vi "SMU Measurement.vi"() -> ()   [LabVIEW 2021]
doc: "Demonstrates how to use the DC Voltage Output Function to force an output voltage. This example initializes a session, configures the Output Function, Sense, Autorange, Voltage Level and Current Limit, initiates generation, waits for a specified delay, and measures the voltage and current output. This example uses Single Point source mode."
uses:
  <instrlib>/niDMM/nidmm.llb/niDMM Resolution in Digits.ctl
  <instrlib>/niDMM/nidmm.llb/niDMM Function.ctl
  <instrlib>/niDCPower/nidcpower.llb/niDCPower Output Function.ctl
  <instrlib>/niDCPower/nidcpower.llb/niDCPower Source Mode.ctl
  <instrlib>/niDMM/nidmm.llb/niDMM Configure Measurement Digits.vi
panel:
  out "SMU Measurement":dbl format="%.6p"
  in  "SMU DMM":refnum<k15>="Dev1"
  in  "SMU DMM Measurement":T1
  out "SMU DMM Resolution":dbl caption="SMU Absolute Resolution" format="%#_3p"
  in  "SMU Resolution in Digits":T2=5.5 items=["3 1/2"=3.5, "4 1/2"=4.5, "5 1/2"=5.5, "6 1/2"=6.5, "7 1/2"=7.5]
  in  "Load SMU":refnum<k15>="Dev1"
  in  "Load SMU Channel":string="0"
  out "Load SMU Current":dbl
  out "Load SMU Voltage":dbl
  in  "error in":errorcluster
  out "error out":errorcluster
  out "Voltage Measurement":dbl caption="Vin SMU Voltage"
  out "Current Measurement":dbl caption="Vin SMU Current"
  in  "Current Limit":dbl=0.01 format="%.3p"
  in  "Voltage Level":dbl=2.0 format="%.5p"
  in  "Vin SMU Channel":string="0"
  in  "Vin SMU":refnum<k15>="Dev1"
  # "Overview: Demonstrates how to use the DC Voltage Output Function to force an output voltage.  \nThis example initializes a session; configures the Output Function, Voltage Level and Current Limit; \ninitiates generation; waits for a specified delay; and measures the voltage and current output. \nRequirements: NI-DCPower\nInstructions:\n1. Select the appropriate device in the Resource Name control.\n2. Configure the parameters of the DC Voltage signal you'd like to output.\n3. Run the VI."
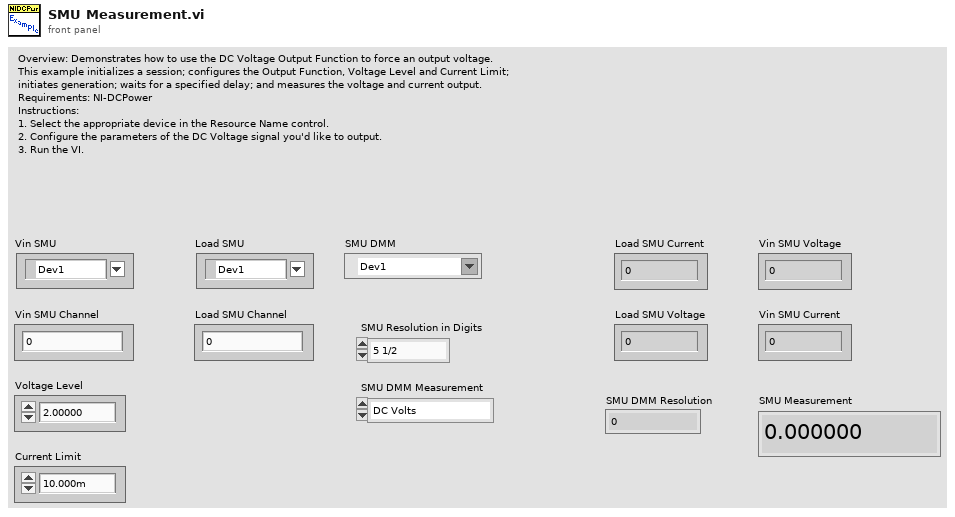
[diagram p1: front panel]
types:
  T1 = typedef "niDMM Function.ctl" = enum16{"DC Volts", "AC Volts", "DC Current", "AC Current", "2-wire Resistance", "4-wire Resistance", "Diode", "Frequency", "Period", "AC Volts DC Coupled", "Capacitance", "Inductance", "Temperature"}
  T2 = typedef "niDMM Resolution in Digits.ctl" = dbl
  T3 = typedef "niDCPower Output Function.ctl" = i32
  T4 = typedef "niDCPower Source Mode.ctl" = i32
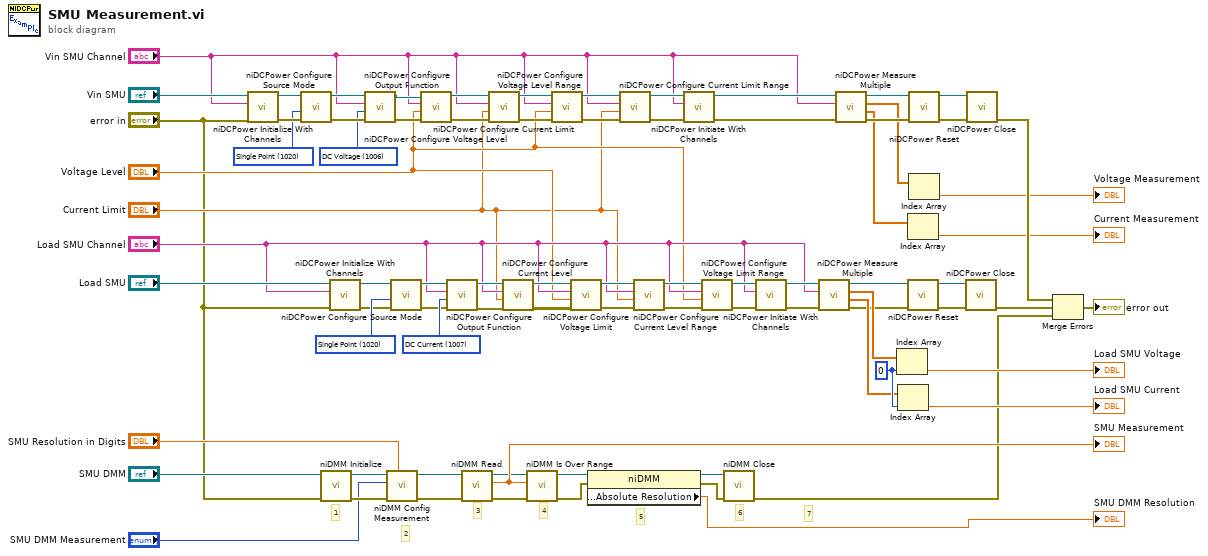
[diagram p0: block diagram]
diagram:
  w51 = T3 1007 items=["DC Voltage"=1006, "DC Current"=1007, "Pulse Voltage"=1049, "Pulse Current"=1050] ("output function")
  w42 = 0 ("index")
  w33 = T4 1020 items=["Single Point"=1020, "Sequence"=1021] ("source mode")
  w57 = T3 1006 items=["DC Voltage"=1006, "DC Current"=1007, "Pulse Voltage"=1049, "Pulse Current"=1050] ("output function")
  w70 = T4 1020 items=["Single Point"=1020, "Sequence"=1021] ("source mode")
  # "2"
  # "1"
  # "7"
  # "6"
  # "5"
  # "4"
  # "3"
  n1 = call <instrlib>:"niDCPower Initialize With Channels.vi"("error in (no error)"="error in", "channels"="Vin SMU Channel", "resource name"="Vin SMU") -> ("error out"=w74:errorcluster, "instrument handle out"=w73:refnum<k15>)  [unwired: 2 in, 5 out]
  n2 = call <instrlib>:"niDCPower Configure Source Mode.vi"("error in (no error)"=w74, "source mode"=w70, "instrument handle"=w73) -> ("error out"=w72:errorcluster, "instrument handle out"=w71:refnum<k15>)  [unwired: 7 out]
  n3 = call <instrlib>:"niDMM Initialize.vi"("error in (no error)"="error in", "Instrument Descriptor"="SMU DMM") -> ("error out"=w10:errorcluster, "instrument handle out"=w11:refnum<k15>)  [unwired: 8 in]
  n4 = call <instrlib>:"niDCPower Initialize With Channels.vi"("error in (no error)"="error in", "channels"="Load SMU Channel", "resource name"="Load SMU") -> ("error out"=w29:errorcluster, "instrument handle out"=w30:refnum<k15>)  [unwired: 2 in, 5 out]
  n5 = call <instrlib>:"niDCPower Configure Output Function.vi"("error in (no error)"=w72, "output function"=w57, "channel name"="Vin SMU Channel", "instrument handle"=w71) -> ("error out"=w58:errorcluster, "instrument handle out"=w59:refnum<k15>)  [unwired: 6 out]
  n6 = call-poly <instrlib>:"niDMM Config Measurement.vi"("Resolution in Digits"="SMU Resolution in Digits", "error in (no error)"=w10, "Function"="SMU DMM Measurement", "instrument handle"=w11) -> ("error out"=w4:errorcluster, "instrument handle out"=w5:refnum<k15>)  [unwired: 6 in]
  n7 = call <instrlib>:"niDCPower Configure Source Mode.vi"("error in (no error)"=w29, "source mode"=w33, "instrument handle"=w30) -> ("error out"=w31:errorcluster, "instrument handle out"=w32:refnum<k15>)  [unwired: 7 out]
  n8 = call <instrlib>:"niDCPower Configure Voltage Level.vi"("error in (no error)"=w58, "voltage level"="Voltage Level", "channel name"="Vin SMU Channel", "instrument handle"=w59) -> ("error out"=w77:errorcluster, "instrument handle out"=w78:refnum<k15>)  [unwired: 6 out]
  n9 = call <instrlib>:"niDCPower Configure Output Function.vi"("error in (no error)"=w31, "output function"=w51, "channel name"="Load SMU Channel", "instrument handle"=w32) -> ("error out"=w49:errorcluster, "instrument handle out"=w50:refnum<k15>)  [unwired: 6 out]
  n10 = call <instrlib>:"niDMM Read.vi"("error in (no error)"=w4, "instrument handle"=w5) -> ("error out"=w7:errorcluster, "Measurement"=w8:dbl, "instrument handle out"=w6:refnum<k15>)  [unwired: 7 in]
  "SMU Measurement" <- w8
  n11 = call <instrlib>:"niDCPower Configure Current Limit.vi"("error in (no error)"=w77, "current limit"="Current Limit", "channel name"="Vin SMU Channel", "instrument handle"=w78) -> ("error out"=w69:errorcluster, "instrument handle out"=w68:refnum<k15>)  [unwired: 1 in, 5 out]
  n12 = call <instrlib>:"niDCPower Configure Current Level.vi"("error in (no error)"=w49, "current level"="Current Limit", "channel name"="Load SMU Channel", "instrument handle"=w50) -> ("error out"=w26:errorcluster, "instrument handle out"=w25:refnum<k15>)  [unwired: 6 out]
  n13 = call <instrlib>:"niDMM Is Over Range.vi"("error in (no error)"=w7, "Measurement"=w8, "instrument handle"=w6) -> ("error out"=w14:errorcluster, "instrument handle out"=w12:refnum<k15>)  [unwired: 6 in, 1 out]
  n14 = call <instrlib>:"niDCPower Configure Voltage Level Range.vi"("error in (no error)"=w69, "voltage level range"="Voltage Level", "channel name"="Vin SMU Channel", "instrument handle"=w68) -> ("error out"=w67:errorcluster, "instrument handle out"=w66:refnum<k15>)  [unwired: 6 out]
  n15 = call <instrlib>:"niDCPower Configure Voltage Limit.vi"("error in (no error)"=w26, "voltage limit"="Voltage Level", "channel name"="Load SMU Channel", "instrument handle"=w25) -> ("error out"=w34:errorcluster, "instrument handle out"=w35:refnum<k15>)  [unwired: 6 out]
  n16 = property class="niDMM"(reference=w12, error in=w14) -> (reference out=w13:refnum<k15>, error out=w15:errorcluster, "Configuration:Absolute Resolution"=→"SMU DMM Resolution":dbl)
  n17 = call <instrlib>:"niDCPower Configure Current Limit Range.vi"("error in (no error)"=w67, "current limit range"="Current Limit", "channel name"="Vin SMU Channel", "instrument handle"=w66) -> ("error out"=w62:errorcluster, "instrument handle out"=w63:refnum<k15>)  [unwired: 6 out]
  n18 = call <instrlib>:"niDCPower Configure Current Level Range.vi"("error in (no error)"=w34, "current level range"="Current Limit", "channel name"="Load SMU Channel", "instrument handle"=w35) -> ("error out"=w36:errorcluster, "instrument handle out"=w37:refnum<k15>)  [unwired: 6 out]
  n19 = call <instrlib>:"niDCPower Initiate With Channels.vi"("error in (no error)"=w62, "channel name"="Vin SMU Channel", "instrument handle"=w63) -> ("error out"=w60:errorcluster, "instrument handle out"=w61:refnum<k15>)  [unwired: 7 in]
  n20 = call <instrlib>:"niDCPower Configure Voltage Limit Range.vi"("error in (no error)"=w36, "voltage limit range"="Voltage Level", "channel name"="Load SMU Channel", "instrument handle"=w37) -> ("error out"=w46:errorcluster, "instrument handle out"=w45:refnum<k15>)  [unwired: 6 out]
  n21 = call <instrlib>:"niDMM Close.vi"("error in (no error)"=w15, "instrument handle"=w13) -> ("error out"=w1:errorcluster)  [unwired: 9 in]
  n22 = call <instrlib>:"niDCPower Initiate With Channels.vi"("error in (no error)"=w46, "channel name"="Load SMU Channel", "instrument handle"=w45) -> ("error out"=w48:errorcluster, "instrument handle out"=w47:refnum<k15>)  [unwired: 7 in]
  n23 = call <instrlib>:"niDCPower Measure Multiple.vi"("error in (no error)"=w48, "channel name"="Load SMU Channel", "instrument handle"=w47) -> ("error out"=w39:errorcluster, "current measurements"=w41:dbl[], "voltage measurements"=w40:dbl[], "instrument handle out"=w38:refnum<k15>)  [unwired: 5 out]
  n24 = call <instrlib>:"niDCPower Measure Multiple.vi"("error in (no error)"=w60, "channel name"="Vin SMU Channel", "instrument handle"=w61) -> ("error out"=w64:errorcluster, "current measurements"=w55:dbl[], "voltage measurements"=w53:dbl[], "instrument handle out"=w65:refnum<k15>)  [unwired: 5 out]
  n25 = Index Array(array=w40, index=w42) -> (element=→"Load SMU Voltage":dbl)
  n26 = Index Array(array=w41, index=w42) -> (element=→"Load SMU Current":dbl)
  n27 = Index Array(array=w55) -> (element=→"Current Measurement":dbl)  [unwired: 1 in]
  n28 = call <instrlib>:"niDCPower Reset.vi"("error in (no error)"=w39, "instrument handle"=w38) -> ("error out"=w28:errorcluster, "instrument handle out"=w27:refnum<k15>)  [unwired: 2 in, 6 out]
  n29 = call <instrlib>:"niDCPower Reset.vi"("error in (no error)"=w64, "instrument handle"=w65) -> ("error out"=w75:errorcluster, "instrument handle out"=w76:refnum<k15>)  [unwired: 2 in, 6 out]
  n30 = Index Array(array=w53) -> (element=→"Voltage Measurement":dbl)  [unwired: 1 in]
  n31 = call <instrlib>:"niDCPower Close.vi"("error in (no error)"=w28, "instrument handle"=w27) -> ("error out"=w22:errorcluster)  [unwired: 9 out]
  n32 = call <instrlib>:"niDCPower Close.vi"("error in (no error)"=w75, "instrument handle"=w76) -> ("error out"=w56:errorcluster)  [unwired: 9 out]
  n33 = Merge Errors(w56, w22, w1) -> (→"error out":errorcluster)
